vi "read.vi"(5 "type to read":refnum<class "Bytes.lvclass">, 9 "length (-1: rest)":i32=-1, 10 "offset (-1: current position)":i32=-1, 11 "Bytes in":refnum<class "Bytes.lvclass">) -> (2 "Bytes read":refnum<class "Bytes.lvclass">, 3 "Bytes out":refnum<class "Bytes.lvclass">)   [LabVIEW 2020, in "lvdata.lvlib" / "Bytes.lvclass"]
uses:
  Bytes.lvclass
  Bytes.lvclass/Bytes.ctl
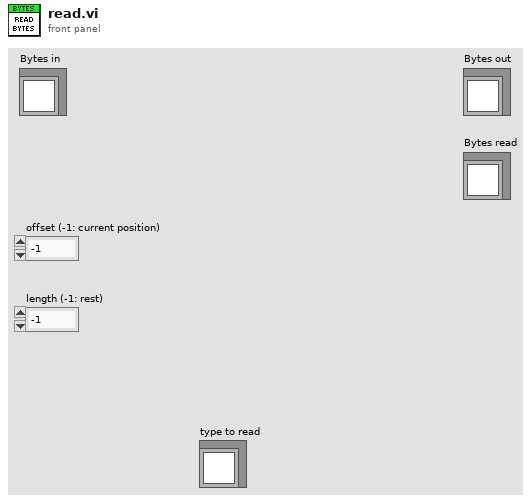
[diagram p1: front panel]
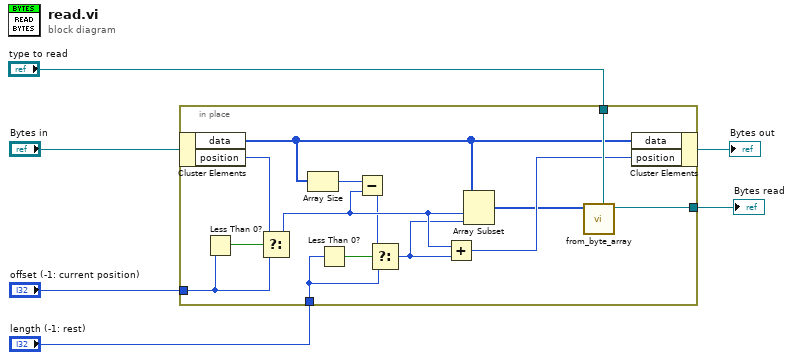
[diagram p0: block diagram]
diagram:
  n1 = in-place {
    in-place-border: "length (-1: rest)" -> [w10]
    in-place-border: "offset (-1: current position)" -> [w16]
    in-place-border: [w20] -> w2
    in-place-border: "type to read" -> [w19]
    n2 = in-place-cluster #1("Bytes in") -> ("data"=w14:u8[], "position"=w17:i32)
    n3 = Less Than 0?(x=w16) -> (x < 0?=w18:bool)
    n4 = Select(t=w17, s=w18, f=w16) -> (s? t:f=w12:i32)
    n5 = Array Size(array=w14) -> (size(s)=w13:i32)
    n6 = Less Than 0?(x=w10) -> (x < 0?=w15:bool)
    n7 = Subtract(x=w13, y=w12) -> (x-y=w11:i32)
    n8 = Select(t=w11, s=w15, f=w10) -> (s? t:f=w9:i32)
    n9 = Add(x=w12, y=w9) -> (x+y=w8:i32)
    n10 = Array Subset(array=w14, index=w12, length=w9) -> (w7:u8[])
    n11 = call "from_byte_array.vi"("type"=w19, "unsigned byte array"=w7) -> ("Bytes out"=w20:refnum<class "Bytes.lvclass">)  [unwired: 9 in]
    n12 = in-place-cluster #1("data"=w14, "position"=w8) -> (→"Bytes out":refnum<class "Bytes.lvclass">)
  }
  "Bytes read" <- w2
